vi "Ball Intake Scaling.vi"(9 "Scaling factor":dbl=0.5, 11 "Intake":bool) -> (3 "IntakeSpeed":dbl)   [LabVIEW 2019]
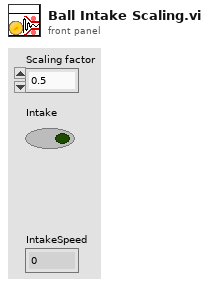
[diagram p1: front panel]
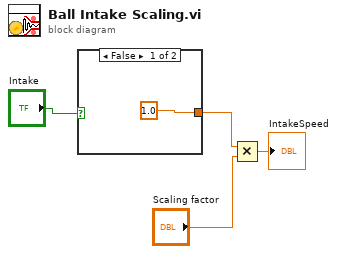
[diagram p0: block diagram]
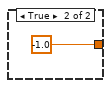
[diagram p2: hidden frame]
diagram:
  n1 = case shown="False" "Intake" {
    tunnel: [1.0 ("x") -1.0 ("x")] -> w1
    frame False {
    }
    frame True {
    }
  }
  n2 = Multiply(x=w1, y="Scaling factor") -> (x*y=→"IntakeSpeed":dbl)
